vi "onDestroy.vi"(8 "error in (no error)":errorcluster, 11 "MQTT_Base in":refnum<class "MQTT_Base.lvclass">) -> (0 "error out":errorcluster, 3 "MQTT_Base out":refnum<class "MQTT_Base.lvclass">)   [LabVIEW 2013, in "MQTT Base.lvlib" / "MQTT_Base.lvclass"]
uses:
  MQTT_Base.lvclass
  MQTT_Base.lvclass/MQTT_Base.ctl
  Subscription/Subscription.lvclass
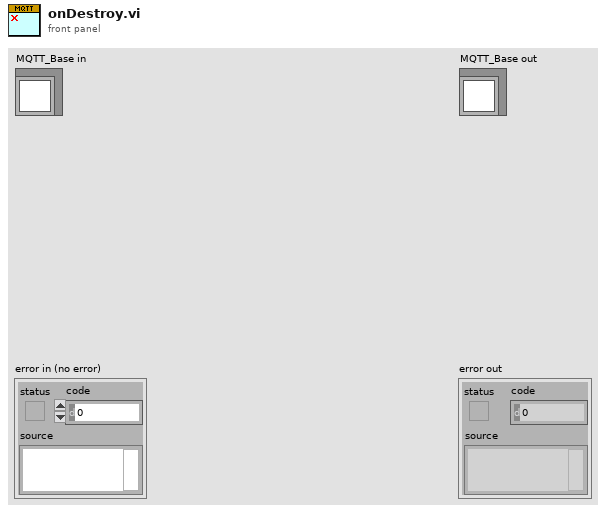
[diagram p1: front panel]
types:
  T1 = typedef "MQTT Base.lvlib/MQTT_Base.lvclass/Public Events -- cluster.ctl" = cluster{"Stop Event":refnum<user-event>, "Error Event":refnum<user-event>, "Inbound Message":refnum<user-event>}
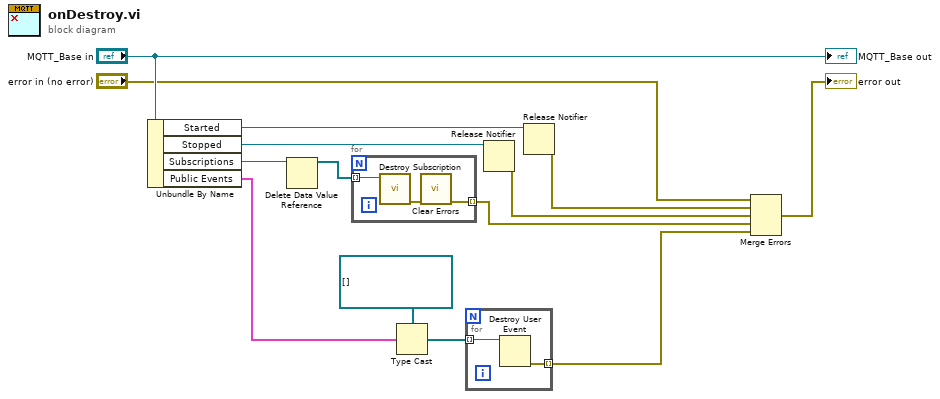
[diagram p0: block diagram]
diagram:
  n1 = Unbundle By Name("MQTT_Base in") -> ("Started"=w8:refnum<notifier>, "Stopped"=w9:refnum<notifier>, "Subscriptions"=w10:refnum<data-value>, "Public Events"=w3:T1)
  n2 = Delete Data Value Reference(data value reference=w10) -> (data value=w11:refnum<class "Subscription.lvclass">[])  [unwired: 1 in, 1 out]
  n3 = for {
    tunnel: w11 -> [w17] mode=indexing
    tunnel: [w15] -> w12 mode=indexing
    n4 = call "Destroy Subscription.vi"("Subscription in"=w17) -> ("error out"=w16:errorcluster)  [unwired: 9 in, 1 out]
    n5 = call <vilib>:"Clear Errors.vi"("error in (no error)"=w16) -> ("error out"=w15:errorcluster)  [unwired: 6 in]
  }
  n6 = Type Cast(type=refnum<user-event>[] [], x=w3) -> (*(type *) &x=w2:refnum<user-event>[])
  n7 = for {
    tunnel: w2 -> [w19] mode=indexing
    tunnel: [w18] -> w1 mode=indexing
    n8 = Destroy User Event(user event=w19) -> (error out=w18:errorcluster)  [unwired: 1 in]
  }
  n9 = Release Notifier(notifier=w9) -> (error out=w14:errorcluster)  [unwired: 2 in, 2 out]
  n10 = Release Notifier(notifier=w8) -> (error out=w13:errorcluster)  [unwired: 2 in, 2 out]
  n11 = Merge Errors("error in (no error)", w13, w14, w12, w1) -> (→"error out":errorcluster)
  "MQTT_Base out" <- "MQTT_Base in"
